vi "VisionAlign.vi"() -> ()   [LabVIEW 2018]
uses:
  Framework/Robot Global Data.vi
panel:
  in  "NoWait":bool
  in  "StoppingDistance":dbl=1.0
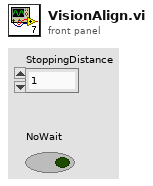
[diagram p1: front panel]
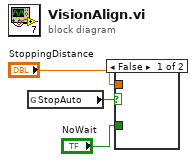
[diagram p0: block diagram]
diagram:
  n1 = global read "Robot Global Data.vi" "StopAuto"() -> (w3:bool)
  n2 = case shown="False" w3 {
    tunnel: "StoppingDistance" -> [_ _]
    tunnel: "NoWait" -> [_ _]
    frame False {
    }
    frame True {
    }
  }
